vi "jsonCreate.vi"(5 "enable extensions?":bool, 7 "allow comments?":bool, 8 "error in (no error)":errorcluster, 10 "json":string) -> (0 "error out":errorcluster, 3 "d":i64)   [LabVIEW 2015, in "rapidjson wrapper.lvlib"]
uses:
  rapidjson wrapper.lvlib
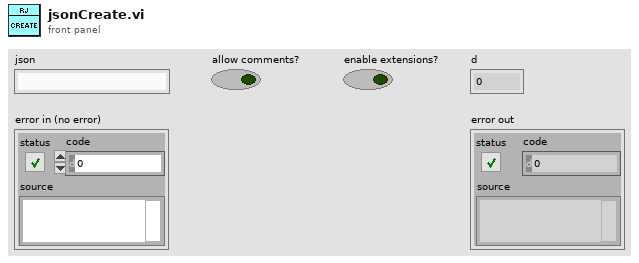
[diagram p1: front panel]
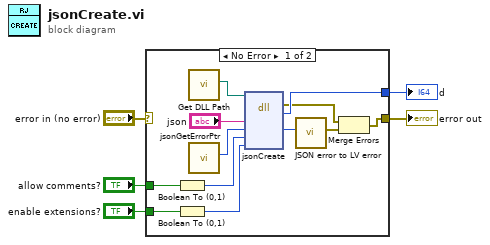
[diagram p0: block diagram]
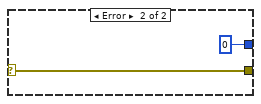
[diagram p2: hidden frame]
diagram:
  n1 = case shown="No Error" "error in (no error)" {
    selector: "error in (no error)" -> [_ w19]
    tunnel: [w15 i64 0 ("return type")] -> w5
    tunnel: [w11 w19] -> w4
    tunnel: "allow comments?" -> [w7 _]
    tunnel: "enable extensions?" -> [w6 _]
    frame No Error {
      n2 = Boolean To (0,1)(Boolean=w7) -> (0, 1=w9:i16)
      n3 = Boolean To (0,1)(Boolean=w6) -> (0, 1=w8:i16)
      n4 = call "Get DLL Path.vi"() -> ("Path"=w10:path)  [unwired: 11 in]
      n5 = call "jsonGetErrorPtr.vi"() -> ("return type"=w16:i64)  [unwired: 10 in, 1 out]
      n6 = dll-call lib="lvrjs*.dll" fn="jsonCreate"(path in=w10, "json"="json", "jsonError"=w16, "allowComments"=w9, "enableExtensions"=w8) -> (error out=w12:errorcluster, "return type"=w15:i64, "jsonError"=w14:i64)  [unwired: 5 in, 1 out]
      n7 = call "JSON error to LV error.vi"("jsonError"=w14) -> ("error out"=w13:errorcluster)  [unwired: 10 in]
      n8 = Merge Errors(w12, w13) -> (w11:errorcluster)
    }
    frame Error {
    }
  }
  "d" <- w5
  "error out" <- w4
